vi "Mangle VI Name__ogtk.vi"   [LabVIEW 2012]
doc: "Mangles a VI's name by applying a <b>namespace string suffix</b>.\n<b>Name</b> may be a path or a string.\nFor example:\n\nName => \"Widget.vi\"\nNamespace => \"OpenG\"\nMangled Name => \"Widget__OpenG.vi\"\n\nName => \"Widget\"\nNamespace => \"OpenG\"\nMangled Name => \"Widget__OpenG\"\n\nName => \"Widget.vi\"\nNamespace => \"\" (Note: blank string means do not mangle)\nMangled Name => \"Widget.vi\""
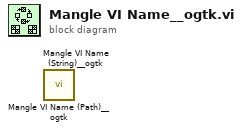
[diagram p0: block diagram]
diagram:
  n1 = call <userlib>:"Mangle VI Name (Path)__ogtk.vi"() -> ()  [unwired: 10 in, 2 out]
  n2 = call <userlib>:"Mangle VI Name (String)__ogtk.vi"() -> ()  [unwired: 10 in, 2 out]
